vi "LMS_FM_Demodulate_Example.vi"() -> ()   [LabVIEW 2018, in "LMS_LV_Drv.lvlib"]
uses:
  LMS_LV_Drv.lvlib
  Stream_ctl.ctl
  <vilib>/sound2/lvsound2.llb/Sampling Mode.ctl
  <vilib>/sound2/lvsound2.llb/Sound Data Format.ctl
  <vilib>/Analysis/3filter.llb/Filter Passband Type.ctl
  <vilib>/Analysis/1siggen.llb/Ramp Pattern by Samples.vi
  <vilib>/Analysis/2dsp.llb/Complex FFT.vi
  <vilib>/sound2/lvsound2.llb/Sound Output Write (DBL Single).vi
  <vilib>/Analysis/3filter.llb/Butterworth Filter (CDB).vi
  <vilib>/Analysis/2dsp.llb/Decimate (continuous, DBL).vi
  <vilib>/Analysis/NI_AALPro.lvlib
  <vilib>/Analysis/NI_AALBase.lvlib
panel:
  out "FM Spectrum":cluster{dbl[], dbl[]}[](graph)
  in  "Direction":u8(ring) items=["RX", "TX"]
  in  "Volume":dbl(knob)=0.14400412422011064 min=0.0 max=2.0 step=0.1 scale=0.0..2.0
  in  "bandwidth":dbl=100000.0 format="%#_6p"
  out "EXIT":bool=TRUE
  in  "stop":bool
  in  "gain":u32
  in  "FM  Frequency":dbl(slide)=100000000.0 min=85000000.0 max=108000000.0 step=50000.0 scale=85000000.0..108000000.0 scale format="%#_6p"
  in  "chan":u64
  in  "stream":T1={"handle"=0, "isTx"=0, "channel"=0, "fifoSize"=100000, "throughputVsLatency"=1.0, "dataFmt"=0}
  out "LimeSDR_info":string="LimeSDR-USB, media=USB 3.0, module=FX3, serial=0009072C02891115, index=0"
  in  "Sample Rate":dbl=2750000.0 format="%#_6p"
  out "error out":errorcluster
  # "FM Demo"
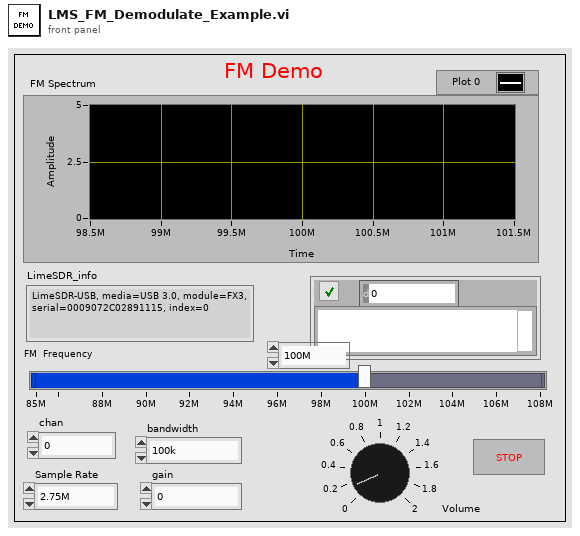
[diagram p1: front panel]
types:
  T1 = typedef "Stream_ctl.ctl" = cluster{"handle":u64, "isTx":u8, "channel":u32, "fifoSize":u32, "throughputVsLatency":dbl, "dataFmt":u32}
  T2 = typedef "Sound Data Format.ctl" = cluster{"sample rate (S/s)":dbl, "number of channels":i32, "bits per sample":i32}
  T3 = typedef "Sampling Mode.ctl" = i32
  T4 = typedef "Sound Output Task ID.ctl" = u32
  T5 = typedef "NI_AALBase.lvlib/Filter Passband Type.ctl" = enum32{"Lowpass", "Highpass", "Bandpass", "Bandstop"}
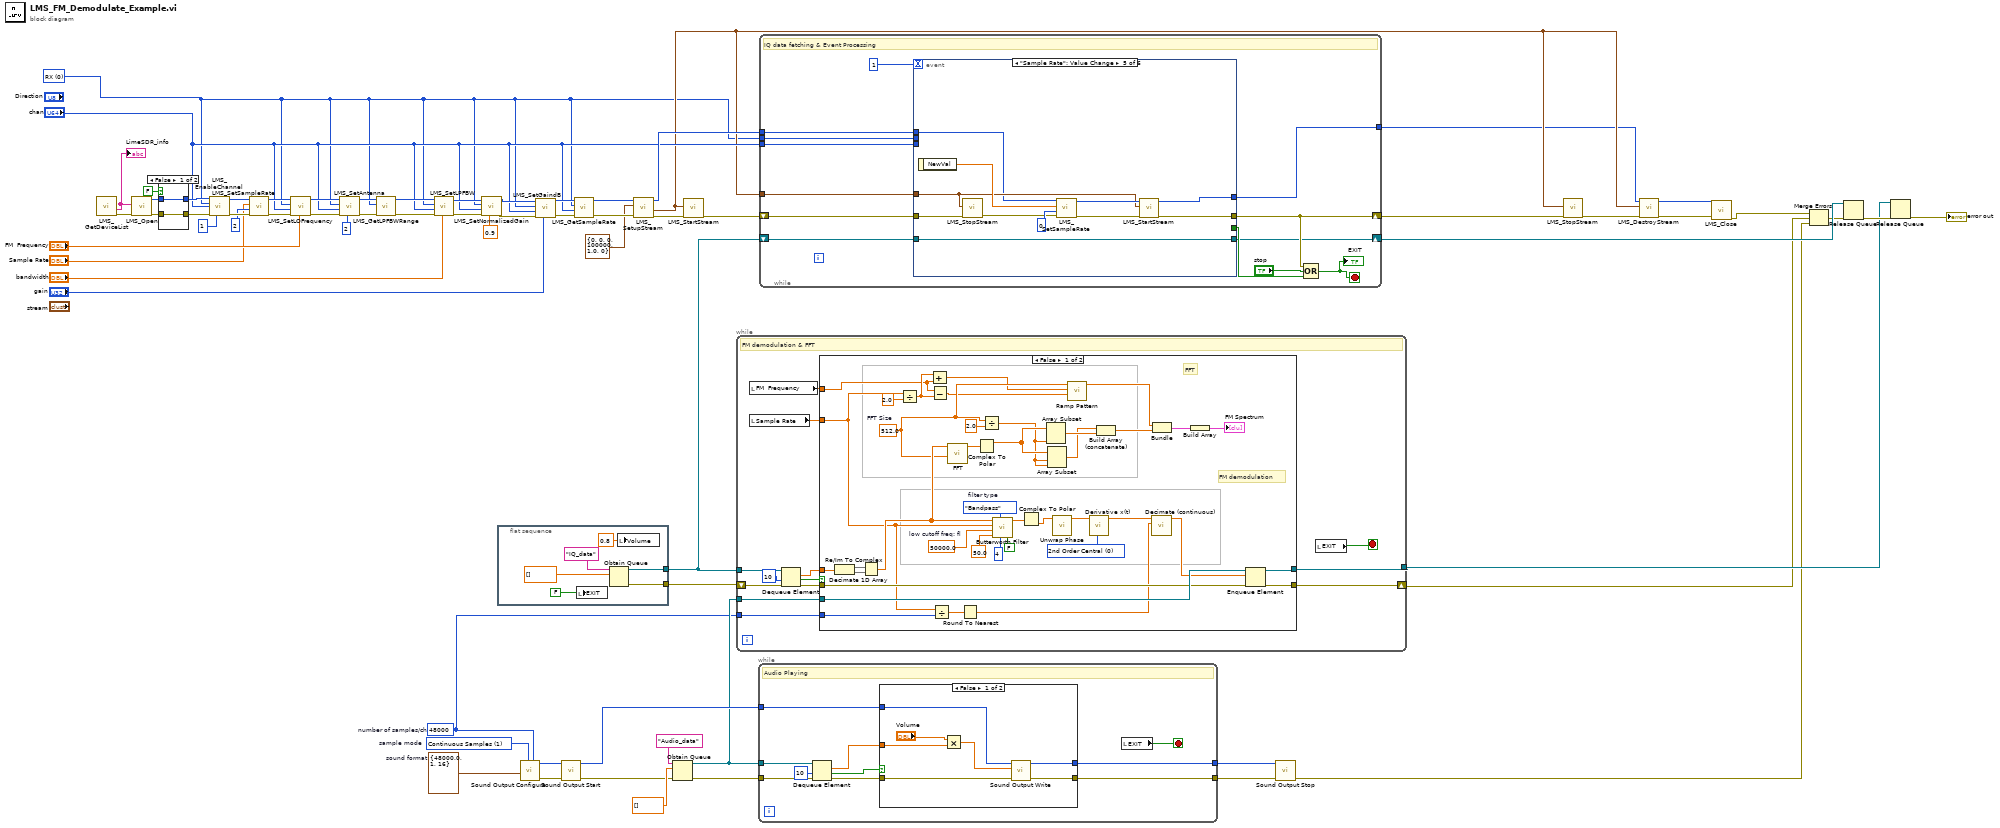
[diagram p0: block diagram]
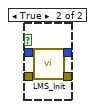
[diagram p2: hidden frame]
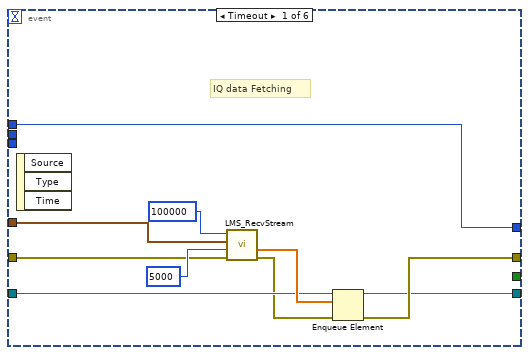
[diagram p5: hidden frame]
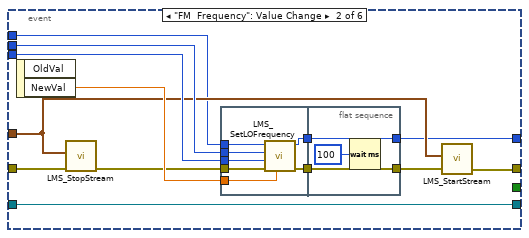
[diagram p6: hidden frame]
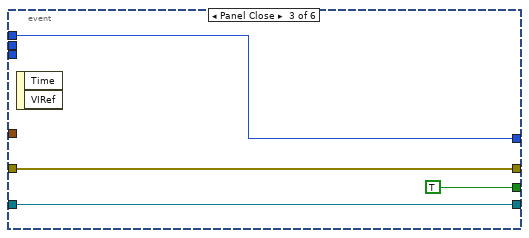
[diagram p7: hidden frame]
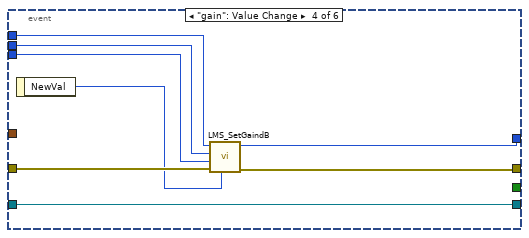
[diagram p8: hidden frame]
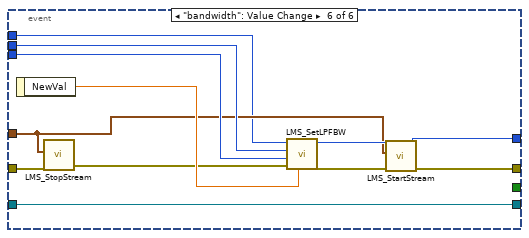
[diagram p9: hidden frame]
diagram:
  w7 = u8 0 items=["RX", "TX"] ("Direction")
  w5 = 48000  # number of samples/ch
  w31 = T2 {"sample rate (S/s)"=48000.0, "number of channels"=1, "bits per sample"=16}  # sound format
  w28 = T3 1 items=["Finite Samples", "Continuous Samples"]  # sample mode
  n1 = call "LMS_GetDeviceList.vi"() -> ("error out"=w68:errorcluster, "lms_info_str_t"=w67:string)  [unwired: 9 in, 1 out]
  "LimeSDR_info" <- w67
  n2 = call "LMS_Open.vi"("error in (no error)"=w68, "lms_info_str_t"=w67) -> ("error out"=w66:errorcluster, "device"=w65:i64)  [unwired: 8 in]
  n3 = case shown="False" FALSE {
    tunnel: w66 -> [w69 w74]
    tunnel: w65 -> [w70 w73]
    tunnel: [w70 w72] -> w56
    tunnel: [w69 w71] -> w55
    frame False {
    }
    frame True {
      n4 = call "LMS_Init.vi"("error in (no error)"=w74, "device_In"=w73) -> ("error out"=w71:errorcluster, "device_Out"=w72:i64)  [unwired: 8 in]
    }
  }
  n5 = call "LMS_EnableChannel.vi"("device_In"=w56, "dir_tx"=w7, "chan"="chan", "error in (no error)"=w55, "enabled"=i8 1) -> ("device_Out"=w52:i64, "error out"=w53:errorcluster)  [unwired: 9 in]
  n6 = call "LMS_SetSampleRate.vi"("error in (no error)"=w53, "oversample"=u64 2, "rate"="Sample Rate", "device_In"=w52) -> ("error out"=w51:errorcluster, "device_Out"=w50:i64)  [unwired: 6 in]
  n7 = call "LMS_SetLOFrequency.vi"("frequency"="FM  Frequency", "error in (no error)"=w51, "chan"="chan", "dir_tx"=w7, "device_In"=w50) -> ("error out"=w46:errorcluster, "device_Out"=w44:i64)  [unwired: 5 in]
  n8 = call "LMS_SetAntenna.vi"("index"=u64 2, "error in (no error)"=w46, "chan"="chan", "dir_tx"=w7, "device_In"=w44) -> ("error out"=w45:errorcluster, "device_Out"=w43:i64)  [unwired: 5 in]
  n9 = call "LMS_GetLPFBWRange.vi"("error in (no error)"=w45, "dir_tx"=w7, "device_In"=w43) -> ("error out"=w48:errorcluster, "device_Out"=w47:i64)  [unwired: 6 in, 1 out]
  n10 = call "LMS_SetLPFBW.vi"("bandwidth"="bandwidth", "error in (no error)"=w48, "chan"="chan", "dir_tx"=w7, "device_In"=w47) -> ("error out"=w41:errorcluster, "device_Out"=w58:i64)  [unwired: 5 in]
  n11 = call "LMS_SetNormalizedGain.vi"("gain"=0.9, "error in (no error)"=w41, "chan"="chan", "dir_tx"=w7, "device_In"=w58) -> ("error out"=w39:errorcluster, "device_Out"=w36:i64)  [unwired: 5 in]
  n12 = flat-sequence {
    tunnel: [w78] -> w37
    tunnel: [w75] -> w2
    frame #0 {
      n13 = local write "EXIT"(FALSE ("EXIT")) -> ()
      n14 = Obtain Queue(name (unnamed)="IQ_data", element data type=dbl[] [] ("samples")) -> (queue out=w78:refnum<queue>, error out=w75:errorcluster)  [unwired: 3 in, 1 out]
      n15 = local write "Volume"(0.8 ("Volume")) -> ()
    }
  }
  n16 = call <vilib>:"Sound Output Configure.vi"("number of samples/ch"=w5, "sample mode"=w28, "sound format"=w31) -> ("error out"=w29:errorcluster, "task ID"=w30:T4)  [unwired: 7 in]
  n17 = call "LMS_SetGaindB.vi"("gain"="gain", "error in (no error)"=w39, "chan"="chan", "dir_tx"=w7, "device_In"=w36) -> ("error out"=w19:errorcluster, "device_Out"=w18:i64)  [unwired: 5 in]
  n18 = call <vilib>:"Sound Output Start.vi"("error in (no error)"=w29, "task ID"=w30) -> ("error out"=w4:errorcluster, "task ID out"=w27:T4)  [unwired: 8 in]
  n19 = call "LMS_GetSampleRate.vi"("error in (no error)"=w19, "chan"="chan", "dir_tx"=w7, "device_In"=w18) -> ("error out"=w59:errorcluster, "device_Out"=w35:i64)  [unwired: 4 in, 2 out]
  n20 = call "LMS_SetupStream.vi"("error in (no error)"=w59, "stream_In"=T1 {"handle"=0, "isTx"=0, "channel"=0, "fifoSize"=100000, "throughputVsLatency"=1.0, "dataFmt"=0} ("stream"), "device_In"=w35) -> ("error out"=w64:errorcluster, "steam_Out"=w9:T1, "device_Out"=w11:i64)  [unwired: 6 in]
  n21 = Obtain Queue(name (unnamed)="Audio_data", element data type=dbl[] [] ("Decimated Array"), error in (no error)=w4) -> (queue out=w15:refnum<queue>, error out=w3:errorcluster)  [unwired: 2 in, 1 out]
  n22 = call "LMS_StartStream.vi"("error in (no error)"=w64, "stream 2"=w9) -> ("error out"=w12:errorcluster)  [unwired: 9 in]
  n23 = while {
    tunnel: w37 -> [w93]
    tunnel: w15 -> [w88]
    tunnel: [w87] -> w33
    shift-right: [w86] -> w23
    shift-left: w2 -> [w85]
    tunnel: w5 -> [w82]
    stop <- w90 stop-if-true
    # "FM demodulation & FFT"
    n24 = local read "FM  Frequency"() -> (w83:dbl)
    n25 = local read "Sample Rate"() -> (w81:dbl)
    n26 = Dequeue Element(queue=w93, timeout in ms (-1)=10, error in (no error)=w85) -> (element=w91:dbl[], timed out?=w92:bool, error out=w84:errorcluster)  [unwired: 1 out]
    n27 = case shown="False" w92 {
      tunnel: w91 -> [w131 _]
      tunnel: w81 -> [w94 _]
      tunnel: w88 -> [w125 w134]
      tunnel: [w124 w134] -> w87
      tunnel: [w123 w133] -> w86
      tunnel: w84 -> [w119 w133]
      tunnel: w83 -> [w100 _]
      tunnel: w82 -> [w96 _]
      frame False {
        w102 = 512.0  # FFT Size
        w126 = u16 0 items=["2nd Order Central", "4th Order Central", "Forward", "Backward"] ("method")
        w127 = Filter_Passband_Type."Bandpass"  # filter type
        w121 = 50000.0  # low cutoff freq: fl
        # "FFT"
        # "FM demodulation"
        n28 = Decimate 1D Array(w131) -> (w130:dbl[], w129:dbl[])
        n29 = Re/Im To Complex(1:w129, 2:w130) -> (0:w114:cdb[])
        n30 = Divide(x=w94, y=2.0) -> (x/y=w101:dbl)
        n31 = Add(x=w101, y=w100) -> (x+y=w98:dbl)
        n32 = Subtract(x=w100, y=w101) -> (x-y=w99:dbl)
        n33 = Divide(x=w94, y=w96) -> (x/y=w97:dbl)
        n34 = call-poly <vilib>:"FFT.vi"("FFT size"=w102, "X"=w114) -> ("FFT {X}"=w132:cdb[])  [unwired: 8 in, 1 out]
        n35 = Round To Nearest(number=w97) -> (nearest integer value=w95:dbl)
        n36 = Complex To Polar(r * e^(i*theta)=w132) -> (r=w110:dbl[])  [unwired: 1 out]
        n37 = Divide(x=w102, y=2.0) -> (x/y=w108:dbl)
        n38 = call-poly <vilib>:"Butterworth Filter.vi"("init/cont (init:F)"=FALSE, "order"=4, "filter type"=w127, "low cutoff freq: fl"=50.0, "high cutoff freq: fh"=w121, "sampling freq: fs"=w94, "X"=w114) -> ("Filtered X"=w113:cdb[])  [unwired: 1 in, 1 out]
        n39 = Complex To Polar(r * e^(i*theta)=w113) -> (theta=w118:dbl[])  [unwired: 1 out]
        n40 = Array Subset(array=w110, length=w108) -> (w112:dbl[])  [unwired: 1 in]
        n41 = Array Subset(array=w110, index=w108, length=w108) -> (w111:dbl[])
        n42 = call <vilib>:"Unwrap Phase.vi"("Phase"=w118) -> ("Unwrapped Phase"=w122:dbl[])  [unwired: 9 in, 1 out]
        n43 = call-poly <vilib>:"Ramp Pattern.vi"("start"=w99, "end"=w98, "samples"=w102) -> ("Ramp Pattern"=w103:dbl[])  [unwired: 7 in, 1 out]
        n44 = call <vilib>:"Derivative x(t).vi"("method"=w126, "X"=w122) -> ("dX/dt"=w117:dbl[])  [unwired: 8 in, 1 out]
        n45 = Build Array (concatenate)(w111, w112) -> (w105:dbl[])
        n46 = call-poly <vilib>:"Decimate (continuous).vi"("decimating factor"=w95, "X"=w117) -> ("Decimated Array"=w115:dbl[])  [unwired: 8 in, 1 out]
        n47 = Bundle("Ramp Pattern"=w103, w105) -> (w107:cluster{"Ramp Pattern":dbl[], dbl[]})  [unwired: 1 in]
        n48 = Build Array(w107) -> (→"FM Spectrum":cluster{"Ramp Pattern":dbl[], dbl[]}[])
        n49 = Enqueue Element(queue=w125, element=w115, error in (no error)=w119) -> (queue out=w124:refnum<queue>, error out=w123:errorcluster)  [unwired: 1 in, 1 out]
      }
      frame True {
      }
    }
    n50 = local read "EXIT"() -> (w90:bool)
  }
  n51 = while {
    tunnel: w15 -> [w142]
    tunnel: w27 -> [w140]
    tunnel: w3 -> [w136]
    tunnel: [w138] -> w26
    tunnel: [w137] -> w25
    stop <- w144 stop-if-true
    # "Audio Playing"
    n52 = Dequeue Element(queue=w142, timeout in ms (-1)=10, error in (no error)=w136) -> (element=w139:dbl[], timed out?=w141:bool, error out=w135:errorcluster)  [unwired: 1 out]
    n53 = case shown="False" w141 {
      tunnel: w140 -> [w148 w153]
      tunnel: w139 -> [w146 _]
      tunnel: w135 -> [w151 w152]
      tunnel: [w150 w152] -> w138
      tunnel: [w149 w153] -> w137
      frame False {
        n54 = Multiply(x="Volume", y=w146) -> (x*y=w147:dbl[])
        n55 = call-poly <vilib>:"Sound Output Write.vi"("error in (no error)"=w151, "data"=w147, "task ID"=w148) -> ("error out"=w150:errorcluster, "task ID out"=w149:T4)  [unwired: 7 in]
      }
      frame True {
      }
    }
    n56 = local read "EXIT"() -> (w144:bool)
  }
  n57 = while {
    tunnel: w9 -> [w162]
    shift-right: [w160] -> w60
    shift-left: w12 -> [w157]
    shift-right: [w154] -> w57
    shift-left: w37 -> [w155]
    tunnel: w11 -> [w166]
    tunnel: w7 -> [w165]
    tunnel: "chan" -> [w164]
    tunnel: [w163] -> w8
    stop <- w161 stop-if-true
    # "IQ data fetching & Event Processing"
    n58 = event shown="[4] \"Sample Rate\": Value Change" {
      selector: _ -> [_ _ _ _ _ _]
      dyn-events: _ -> [_ _ _ _ _ _]
      timeout: u32 1 ("milliseconds to wait") -> [_ _ _ _ _ _]
      tunnel: w157 -> [w173 w186 w203 w211 w218 w227]
      tunnel: w166 -> [w171 w177 w202 w209 w215 w223]
      tunnel: [w171 w182 w202 w208 w220 w231] -> w163
      tunnel: [w168 w185 w203 w210 w216 w225] -> w160
      tunnel: w165 -> [_ w189 _ w207 _ w230]
      tunnel: w164 -> [_ w188 _ w206 _ w229]
      tunnel: [_ _ TRUE _ _ _] -> w158
      tunnel: w162 -> [w172 w183 _ _ w217 w224]
      tunnel: w155 -> [w170 w184 w200 w204 w219 w228]
      tunnel: [w167 w184 w200 w204 w219 w228] -> w154
      event Timeout {
        # "IQ data Fetching"
        n59 = event-data() -> ()  [unwired: 1 in, 3 out]
        n60 = call "LMS_RecvStream.vi"("error in (no error)"=w173, "timeout_ms"=u32 5000, "stream"=w172, "sample_count"=u64 100000) -> ("error out"=w169:errorcluster, "samples"=w176:dbl[])  [unwired: 6 in]
        n61 = Enqueue Element(queue=w170, element=w176, error in (no error)=w169) -> (queue out=w167:refnum<queue>, error out=w168:errorcluster)  [unwired: 1 in, 1 out]
      }
      event "FM  Frequency": Value Change {
        n62 = event-data() -> ("NewVal"=w187:dbl)  [unwired: 1 in, 1 out]
        n63 = call "LMS_StopStream.vi"("error in (no error)"=w186, "stream"=w183) -> ("error out"=w178:errorcluster)  [unwired: 9 in]
        n64 = flat-sequence {
          tunnel: w189 -> [w196]
          tunnel: w188 -> [w195]
          tunnel: w187 -> [w194]
          tunnel: w178 -> [w193]
          tunnel: w177 -> [w192]
          tunnel: [w191] -> w180
          tunnel: [w190] -> w179
          tunnel: [w198] -> w181
          tunnel: [w199] -> w182
          tunnel: w180 -> [w199]
          tunnel: w179 -> [w198]
          frame #0 {
            n65 = call "LMS_SetLOFrequency.vi"("frequency"=w194, "error in (no error)"=w193, "chan"=w195, "dir_tx"=w196, "device_In"=w192) -> ("error out"=w190:errorcluster, "device_Out"=w191:i64)  [unwired: 5 in]
          }
          frame #1 {
            n66 = Wait (ms)(milliseconds to wait=u32 100) -> ()  [unwired: 1 out]
          }
        }
        n67 = call "LMS_StartStream.vi"("error in (no error)"=w181, "stream 2"=w183) -> ("error out"=w185:errorcluster)  [unwired: 9 in]
      }
      event Panel Close {
        n68 = event-data() -> ()  [unwired: 1 in, 2 out]
      }
      event "gain": Value Change {
        n69 = event-data() -> ("NewVal"=w205:u32)  [unwired: 1 in]
        n70 = call "LMS_SetGaindB.vi"("gain"=w205, "error in (no error)"=w211, "chan"=w206, "dir_tx"=w207, "device_In"=w209) -> ("error out"=w210:errorcluster, "device_Out"=w208:i64)  [unwired: 5 in]
      }
      event "Sample Rate": Value Change {
        n71 = event-data() -> ("NewVal"=w221:dbl)  [unwired: 1 in]
        n72 = call "LMS_StopStream.vi"("error in (no error)"=w218, "stream"=w217) -> ("error out"=w212:errorcluster)  [unwired: 9 in]
        n73 = call "LMS_SetSampleRate.vi"("error in (no error)"=w212, "oversample"=u64 0, "rate"=w221, "device_In"=w215) -> ("error out"=w213:errorcluster, "device_Out"=w220:i64)  [unwired: 6 in]
        n74 = call "LMS_StartStream.vi"("error in (no error)"=w213, "stream 2"=w217) -> ("error out"=w216:errorcluster)  [unwired: 9 in]
      }
      event "bandwidth": Value Change {
        n75 = event-data() -> ("NewVal"=w232:dbl)  [unwired: 1 in]
        n76 = call "LMS_StopStream.vi"("error in (no error)"=w227, "stream"=w224) -> ("error out"=w222:errorcluster)  [unwired: 9 in]
        n77 = call "LMS_SetLPFBW.vi"("bandwidth"=w232, "error in (no error)"=w222, "chan"=w229, "dir_tx"=w230, "device_In"=w223) -> ("error out"=w226:errorcluster, "device_Out"=w231:i64)  [unwired: 5 in]
        n78 = call "LMS_StartStream.vi"("error in (no error)"=w226, "stream 2"=w224) -> ("error out"=w225:errorcluster)  [unwired: 9 in]
      }
    }
    n79 = Compound Arithmetic op=OR(w160, "stop", w158) -> (w161:bool)
    "EXIT" <- w161
  }
  n80 = call <vilib>:"Sound Output Stop.vi"("error in (no error)"=w26, "task ID"=w25) -> ("error out"=w22:errorcluster)  [unwired: 8 in, 1 out]
  n81 = call "LMS_StopStream.vi"("error in (no error)"=w60, "stream"=w9) -> ("error out"=w61:errorcluster)  [unwired: 9 in]
  n82 = call "LMS_DestroyStream.vi"("error in (no error)"=w61, "stream"=w9, "device_In"=w8) -> ("error out"=w63:errorcluster, "device_Out"=w62:i64)  [unwired: 7 in]
  n83 = call "LMS_Close.vi"("error in (no error)"=w63, "device_In"=w62) -> ("error out"=w24:errorcluster)  [unwired: 9 in]
  n84 = Merge Errors(w24, w23, w22) -> (w21:errorcluster)
  n85 = Release Queue(queue=w57, error in (no error)=w21) -> (error out=w34:errorcluster)  [unwired: 1 in, 2 out]
  n86 = Release Queue(queue=w33, error in (no error)=w34) -> (error out=→"error out":errorcluster)  [unwired: 1 in, 2 out]
